vi "FOV.vi"(11 "Camera view angles":dbl[][](array[numeric])=[[51.7, 49.4, 64.0, 49.2, 60.0], [32.0, 30.0, 38.0, 35.1, 35.0], [61.0, 58.0, 74.4, 61.0, 69.4]]) -> (3 "FOV":dbl=41.0, 10 "Camera view angles 2":dbl[](array[numeric])=[51.7, 49.4, 64.0, 52.0, 41.0])   [LabVIEW 2020]
uses:
  Get camera FOVs Folder/Camera Types.ctl
panel:
  in  "Type":enum16{"Horizontal", "Vertical", "Diagonal"}(ring)
  in  "Camera Type":T1
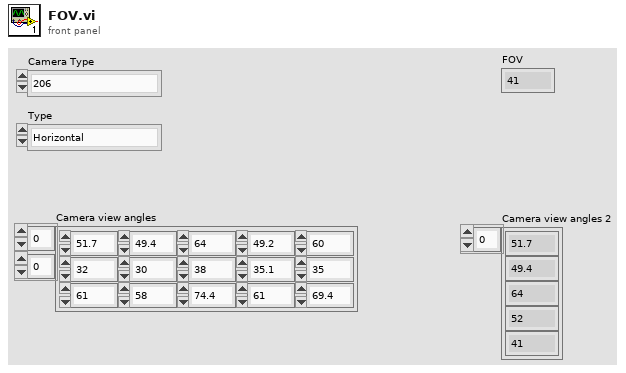
[diagram p1: front panel]
types:
  T1 = typedef "Camera Types.ctl" = enum16{"206", "1011", "1013", "MS HD3000 square", "MS HD3000 640x480"}
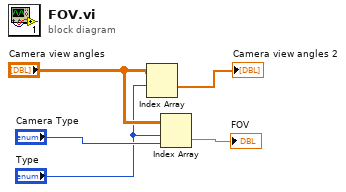
[diagram p0: block diagram]
diagram:
  n1 = Index Array(array="Camera view angles", index (row)="Type") -> (element=→"Camera view angles 2":dbl[])  [unwired: 1 in]
  n2 = Index Array(array="Camera view angles", index (row)="Type", index (col)="Camera Type") -> (element=→"FOV":dbl)
